vi "Climb Loop.vi"   [LabVIEW 2016]
uses:
  Common Code/Utilities/Change Detect Boolean.vi
  Robot Global Data.vi
types:
  T1 = typedef "Dashboard Control Data.ctl" = cluster{"Drivetrain Settings":T2, "Intake Presets ":T4, "Shooter Presets":T5, "Vision Target Packet":T6, "Auton Presets":cluster{"Start Position":dbl}, "Drivetrain Encoder Values":T7, "Drivetrain Encoder Settings":cluster{"Left Tick Constant":dbl, "Right Tick Contant":dbl, "Reset Encoders":bool, "Center Tick Constant":dbl}, "Zero Gyro":bool, "Vision Timeout":dbl, "Pressure M":dbl, "Pressure B":dbl, "Auto Agitator":T9, "Climber Settings":T10}
  T2 = typedef "Drivetrain Settings.ctl" = cluster{"Gyro Tolerance":dbl, "Gyro Steer PID Gains":T3, "Y Power Multiplier":dbl, "Turn Power Multiplier":dbl, "Gyro Output":dbl, "Creep Rate":dbl, "Distance Drive PID Gains":T3, "Distance Tolerance":dbl, "Distance Output":dbl, "Strafe Threshold":dbl, "Strafe Correct":bool, "Strafe Corect Tolerance":dbl, "Translate Drive PID Gains":T3, "Strafe Output":dbl, "SC Right":dbl, "SC Left":dbl, "Use Gyro":bool, "Constant Power":bool, "Strafe Power":dbl}
  T3 = typedef "PID Gains.ctl" = cluster{"proportional gain (Kc)":dbl, "integral time (Ti, min)":dbl, "derivative time (Td, min)":dbl}
  T4 = typedef "Intake Presets.ctl" = cluster{"Intake Speed ":dbl, "Outake Speed":dbl, "Current Trip Delay":dbl, "Max Current":dbl, "Gear Outtake Motor Dellay":dbl}
  T5 = typedef "Shooter Presets.ctl" = cluster{"Key Shot":cluster{"RPM ":dbl, "Hood?":bool}, "Distance Shot":cluster{"RPM":dbl, "Hood?":bool}, "RPM Tolerance":dbl, "Unstuck Delay Time ":dbl, "Initial RPM Increase":dbl, "Warmup Delay":dbl, "Faster Time":dbl, "Shooter PID Gains":cluster{"P":dbl, "I":dbl, "D":dbl, "FF":dbl, "Ramp Rate":dbl, "I Zone":dbl}, "Unstuck Trigger Power":dbl, "Trigger Power":dbl, "Unstuck RPM":dbl, "Agitator Active Power":dbl, "Agitator Idle Power":dbl}
  T6 = typedef "Vision Target Packet.ctl" = cluster{"Robot Center":dbl, "Center X":dbl, "Center Y":dbl, "Angle":dbl, "Distance":dbl, "Found Target?":bool}
  T7 = typedef "Drivetrain Encoder Values.ctl" = cluster{"Left Encoder":T8, "Center Encoder":T8, "Right Encoder":T8}
  T8 = typedef "Encoder Values.ctl" = cluster{"Distance":dbl, "Speed":dbl, "Tick":dbl}
  T9 = typedef "Auto Agitator Settings.ctl" = cluster{"Enable Auto Agitation":bool, "Continuous Stir":bool, "Continuous Intake":bool, "Alternate In/Outtake":bool, "Wing Delay":dbl, "Stir Delay":dbl, "Intake Delay":dbl, "Wing On Time":dbl, "Wing Off Time":dbl, "Stir On Time":dbl, "Stir Off Time":dbl, "Intake On Time":dbl, "Intake Off Time":dbl, "Stir Power":dbl, "Intake Power":dbl, "Outtake Power":dbl, "Intake Run Time":dbl, "Outtake Run Time":dbl, "Wing$":bool, "Intake":bool, "Stirrer":bool}
  T10 = typedef "Climber Settings.ctl" = cluster{"Climber Power":dbl, "Max Current":dbl, "Avoid Current Trip?":bool}
  T11 = typedef "Climb Command Cluster.ctl" = cluster{"Go Up":bool}
  T12 = typedef "WPI_MotorControlDeviceRef.ctl" = cluster{"DeviceStatus":errorcluster, "Type":T13, "PWM":cluster{"PWM Channel":T14, "DeadBand":T15}, "CAN":cluster{"Device Number":u8, "SetOutput VI Ref":variant, "GetOutput VI Ref":variant, "Enable VI Ref":variant, "Disable VI Ref":variant, "Data":variant}, "Invert":bool}
  T13 = typedef "WPI_MotorControlType.ctl" = enum16{"PWM", "CAN"}
  T14 = typedef "FPGA_DIOPWMChannel.ctl" = enum8{"PWM 0", "PWM 1", "PWM 2", "PWM 3", "PWM 4", "PWM 5", "PWM 6", "PWM 7", "PWM 8", "PWM 9", "PWM MXP 0", "PWM MXP 1", "PWM MXP 2", "PWM MXP 3", "PWM MXP 4", "PWM MXP 5", "PWM MXP 6", "PWM MXP 7", "PWM MXP 8", "PWM MXP 9", "Invalid"}
  T15 = typedef "WPI_PWMDeadband.ctl" = cluster{"Name":string, "maxPositivePwm":i32, "minPositivePwm":i32, "centerPwm":i32, "maxNegativePwm":i32, "minNegativePwm":i32, "angularRange":u16}
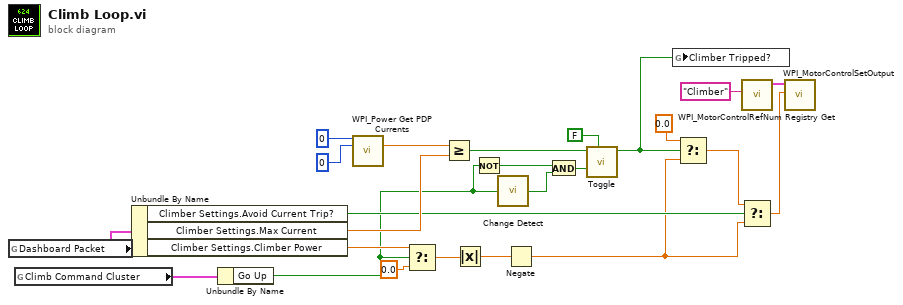
[diagram p0: block diagram]
diagram:
  n1 = global read "Robot Global Data.vi" "Dashboard Packet"() -> (w19:T1)
  n2 = global read "Robot Global Data.vi" "Climb Command Cluster"() -> (w21:T11)
  n3 = Unbundle By Name(w19) -> ("Climber Settings.Avoid Current Trip?"=w12:bool, "Climber Settings.Max Current"=w13:dbl, "Climber Settings.Climber Power"=w18:dbl)
  n4 = Unbundle By Name(w21) -> ("Go Up"=w7:bool)
  n5 = call <vilib>:"WPI_Power Get PDP Currents.vi"("Power Distribution Panel (0)"=u8 0, "PDP Channel"=0) -> ("current (A)"=w14:dbl)  [unwired: 11 in, 2 out]
  n6 = Select(t=w18, s=w7, f=0.0) -> (s? t:f=w20:dbl)
  n7 = Greater Or Equal?(x=w14, y=w13) -> (x >= y?=w8:bool)
  n8 = Absolute Value(x=w20) -> (abs(x)=w17:dbl)
  n9 = Not(x=w7) -> (.not. x?=w6:bool)
  n10 = call-poly "Change Detect.vi"("In"=w7) -> ("Changed?"=w9:bool)
  n11 = Negate(x=w17) -> (-x=w2:dbl)
  n12 = And(x=w6, y=w9) -> (x .and. y?=w5:bool)
  n13 = call "Toggle.vi"("Reinit?"=w5, "Initial Value"=FALSE, "In"=w8) -> ("Toggled"=w1:bool)  [unwired: 8 in]
  n14 = global write "Robot Global Data.vi" "Climber Tripped?"(w1) -> ()
  n15 = Select(t=0.0, s=w1, f=w2) -> (s? t:f=w3:dbl)
  n16 = call <vilib>:"WPI_MotorControlRefNum Registry Get.vi"("refnum name"="Climber") -> ("MotorControlDevRef"=w24:T12)  [unwired: 9 in, 1 out]
  n17 = Select(t=w3, s=w12, f=w2) -> (s? t:f=w11:dbl)
  n18 = call <vilib>:"WPI_MotorControlSetOutput.vi"("Output"=w11, "MotorControlDevRef"=w24) -> ()  [unwired: 7 in, 3 out]
